vi "Set Fill Mode.vi"(8 "error in (no error)":errorcluster, 10 "Fill Mode":T1="ON", 11 "Instrument.1820 in":refnum<class "Instrument.Oxford1820.lvclass">) -> (0 "error out":errorcluster, 3 "Instrument.1820 in":refnum<class "Instrument.Oxford1820.lvclass">)   [LabVIEW 2016, in "Instrument.Oxford1820.lvclass"]
uses:
  Instrument.Oxford1820.lvclass
  <instrlib>/Mercury iXX/Public/Libraries/Magnet/Controls/Fill Mode-Combo.ctl
  Typedefs/Instrument.Oxford1820.Commands-enum.ctl
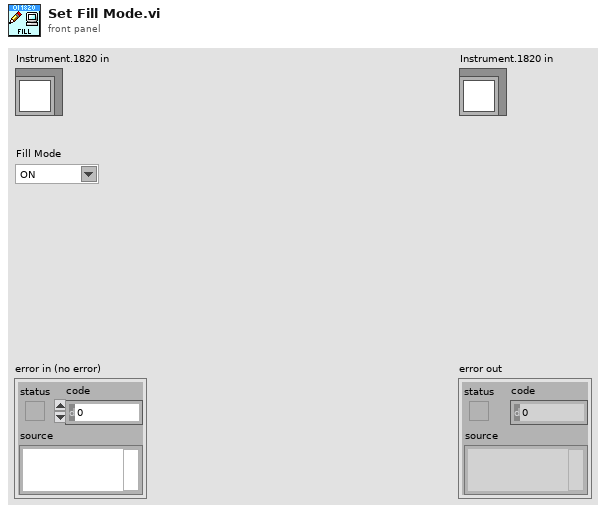
[diagram p1: front panel]
types:
  T1 = typedef "Instrument.Oxford1820.lvclass/Fill Mode-Combo.ctl" = string
  T2 = typedef "Instrument.Oxford1820.lvclass/Instrument.Oxford1820.Commands-enum.ctl" = enum16{"setAction", "setTarget", "setSwitchHeat", "setLambda", "setFillMode", "setNeedleValve", "setMagnetField", "getStatus", "getTarget", "getSwitchHeat", "getPSUField", "getMagnetField"}
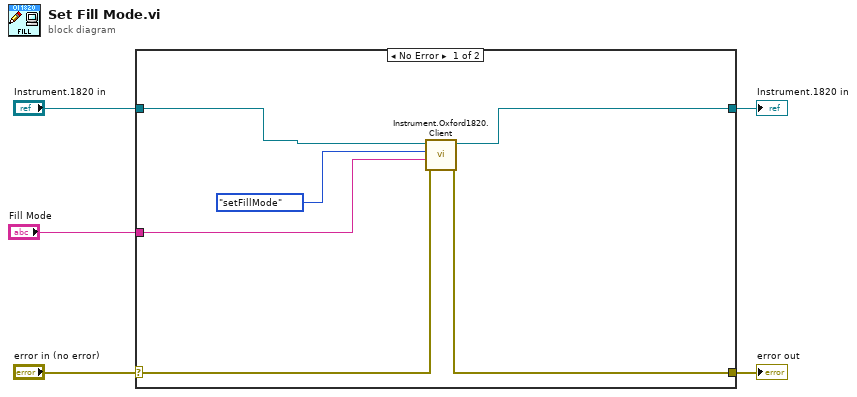
[diagram p0: block diagram]
diagram:
  n1 = case shown="No Error" "error in (no error)" {
    selector: "error in (no error)" -> [w10 w13]
    tunnel: [w9 w13] -> w4
    tunnel: [w6 w12] -> w2
    tunnel: "Instrument.1820 in" -> [w7 w12]
    tunnel: "Fill Mode" -> [w8 _]
    frame No Error {
      n2 = call "Instrument.Oxford1820.Client.vi"("error in (no error)"=w10, "Data"=w8, "Commands"=Instrument.Oxford1820.Commands-enum."setFillMode", "Instrument.1820 in"=w7) -> ("error out"=w9:errorcluster, "Instrument.1820 out"=w6:refnum<class "Instrument.Oxford1820.lvclass">)  [unwired: 5 in, 1 out]
    }
    frame Error {
    }
  }
  "error out" <- w4
  "Instrument.1820 in" <- w2
